vi "read_config_file.vi"(8 "error in (no error)":errorcluster, 10 "force load?":bool, 11 "YK090817SutterMP285Stage in":refnum<class "YK090817SutterMP285Stage.lvclass">=refnum) -> (0 "error out":errorcluster, 3 "YK090817SutterMP285Stage out":refnum<class "YK090817SutterMP285Stage.lvclass">)   [LabVIEW 2010, in "YK090817SutterMP285Stage.lvclass"]
doc: "The dynamic dispatch version of this VI loads the config file from the config_files folder of the actual plug-in class. The name of the config file to be loaded is property of the plug-in object. If not explicitely set, a file config_files/config.xml is loaded by default."
uses:
  YK090817SutterMP285Stage.lvclass
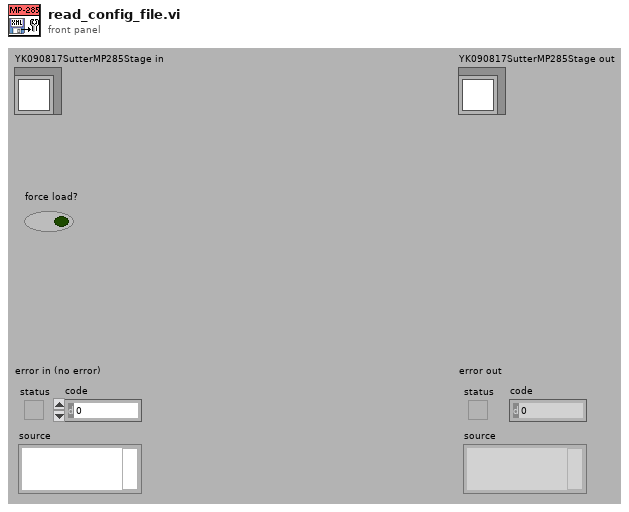
[diagram p1: front panel]
types:
  T1 = cluster{"serial port":i8, "HiRes Speed":dbl, "LoRes Speed":dbl}
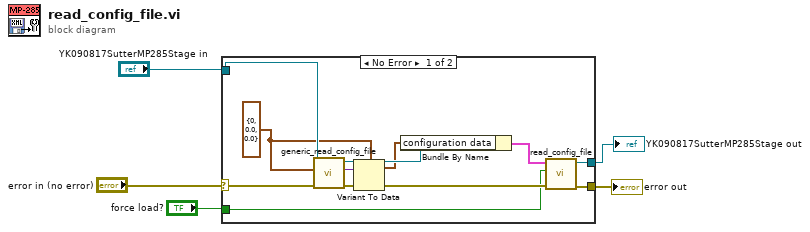
[diagram p0: block diagram]
diagram:
  n1 = case shown="No Error" "error in (no error)" {
    selector: "error in (no error)" -> [w14 w18]
    tunnel: [w17 w18] -> w2
    tunnel: [w16 w19] -> w4
    tunnel: "YK090817SutterMP285Stage in" -> [w12 w19]
    tunnel: "force load?" -> [w6 _]
    frame No Error {
      w7 = T1 {"serial port"=0, "HiRes Speed"=0.0, "LoRes Speed"=0.0} ("configuration data")
      n2 = call-dynamic "generic_read_config_file.vi"("error in (no error)"=w14, "config cluster variant in (data type)"=w7, "GenericPlugin in"=w12) -> ("error out"=w15:errorcluster, "config cluster variant out (populated"=w11:variant, "GenericPlugin out"=w10:refnum<class "YK090817SutterMP285Stage.lvclass">)  [unwired: 6 out]
      n3 = Variant To Data(error in=w15, Variant=w11, type=w7) -> (error out=w13:errorcluster, data=w8:T1)
      n4 = Bundle By Name(cluster=w10, "configuration data"=w8) -> (w9:cluster{})
      n5 = call-parent "read_config_file.vi"("error in (no error)"=w13, "force load?"=w6, "GenericPlugin in"=w9) -> ("error out"=w17:errorcluster, "GenericPlugin out"=w16:refnum<class "YK090817SutterMP285Stage.lvclass">)  [unwired: 7 out]
    }
    frame Error {
    }
  }
  "error out" <- w2
  "YK090817SutterMP285Stage out" <- w4
